vi "Define Abstractly.vi"(10 "Relation Definition":T1={"Type"={"Name"="", "Nullable"=FALSE, "Default NULL"=FALSE}, "Relation"={"Mapping"=enum."OneToMany", "Related To"="", "Reversed By"=""}}, 11 "Relation in":refnum<class "Relation.lvclass">) -> (3 "Relation out":refnum<class "Relation.lvclass">)   [LabVIEW 2020, in "Conditu2.lvlib" / "Columns.lvlib" / "Relation.lvclass"]
uses:
  Relation.lvclass
  C:/dev/lv20CE/lv-conditum-tools/Conditum-Clone/Columns/Type/Type.lvclass
  Relation Definition.ctl
  Type/Definition.ctl
  Relation Info.ctl
  Relation Mapping.ctl
  Type/Type.lvclass/Type.ctl
  Relation.lvclass/Relation.ctl
  Type/Define Type.vi
  Type/Type.lvclass
  Conditu2.lvlib
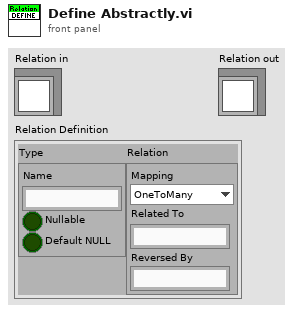
[diagram p1: front panel]
types:
  T1 = typedef "Conditu2.lvlib/Columns.lvlib/Relation.lvclass/Relation Definition.ctl" = cluster{"Type":T2, "Relation":T3}
  T2 = typedef "Conditu2.lvlib/Columns.lvlib/Type.lvclass/Definition.ctl" = cluster{"Name":string, "Nullable":bool, "Default NULL":bool}
  T3 = typedef "Conditu2.lvlib/Relation Info.ctl" = cluster{"Mapping":T4, "Related To":string, "Reversed By":string}
  T4 = typedef "Conditu2.lvlib/Relation Mapping.ctl" = enum16{"OneToOne", "OneToMany", "ManyToOne", "ManyToMany"}
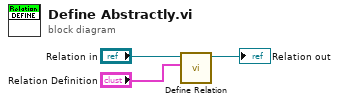
[diagram p0: block diagram]
diagram:
  n1 = call "Define Relation.vi"("Relation Definition"="Relation Definition", "Relation in"="Relation in") -> ("Relation out"=→"Relation out":refnum<class "Relation.lvclass">)  [unwired: 9 in]
